vi "ADQUIRI_adq.vi"() -> ()   [LabVIEW 2019]
doc: "Programa que faz a leitura e a gravação em arquivo TXT de 13 canais provenientes da placa da National Instruments."
uses:
  <vilib>/DAQmx/read.llb/DAQmx Read (Analog 2D DBL NChan NSamp).vi
  <vilib>/Analysis/baseanly.llb/Mean (DBL).vi
  comunicacao.vi
  Aplicacao_atual_global_adq.vi
  <vilib>/DAQmx/configure/timing.llb/DAQmx Timing (Sample Clock).vi
  <vilib>/DAQmx/miscellaneous.llb/DAQmx Fill In Error Info.vi
  <vilib>/Utility/file.llb/Write Delimited Spreadsheet (DBL).vi
  <vilib>/Analysis/NI_AALBase.lvlib
  <vilib>/Utility/file.llb/Read Delimited Spreadsheet (string).vi
  <vilib>/Utility/file.llb/Write Delimited Spreadsheet (string).vi
panel:
  in  "JK(N. Arquivo)":string
  in  "JW(N. Arquivo)":string
  out "data path":path
  out "arrayPbar":dbl[](array[numeric])
  out "Pbarometro":dbl format="%#.2g"
  in  "JG(N. Arquivo)":string
  out "P1-P2 VERDE":bool
  out "comunica funcionando":bool
  in  "Calibração":bool
  in  "COMUNICA":bool
  out "DAQmx Task Name":refnum<k21>
  in  "Visualizar":bool
  out "led viewing":bool
  out "Configuração":string
  in  "Pontos No Gráfico":dbl(knob)=497.5700948522667 scale=0.0..3000.0
  in  "Frequência":dbl=3000.0
  out "Ok":bool
  out "OK2":bool
  out "Ok R":bool
  out "OK2 R":bool
  out "SKM-AI-KF-COR":dbl
  out "SKM-FI-WF":dbl format="%#.2g"
  out "SKM-FIC-KF-COR":dbl format="%#.2g"
  in  "SAIR":bool
  out "JG(m/s)":dbl
  in  "TempoAquisicao":dbl=60.0
  out "JW(m/s)":dbl format="%#.6g"
  out "JK(m/s)":dbl format="%#.6g"
  out "Timer":i32 caption="Elapsed Time (s)"
  in  "COMEÇAR":bool
  out "Quantidade de\narquivos adquiridos":i64
  out "LED adquiri":bool
  out "Aquisição Automática":bool
  out "Linha de Teste":bool
  in  "Tab Control":enum32{"Gráfico", "Matriz"}(tab)
  out "Aplicação":string
  in  "Help":bool
  out "Gráfico":dbl[][](graph)
  out "C1-M corrente":dbl format="%#_4g"
  out "C1-J corrente":dbl format="%#_4g"
  out "C2-M corrente":dbl format="%#_4g"
  out "C2-J corrente":dbl format="%#_4g"
  out "C3-M corrente":dbl format="%#_4g"
  out "C3-J corrente":dbl format="%#_4g"
  out "C4-M corrente":dbl format="%#_4g"
  out "C4-J corrente":dbl format="%#_4g"
  out "P1 corrente":dbl format="%#_4g"
  out "P2 corrente":dbl format="%#_4g"
  out "P3 corrente":dbl format="%#_4g"
  out "P4 corrente":dbl format="%#_4g"
  out "Pfundo corrente":dbl format="%#_4g"
  out "P4(kPa)":dbl format="%#.2g"
  out "P3(kPa)":dbl format="%#.2g"
  out "P2(kPa)":dbl format="%#.2g"
  out "P1(kPa)":dbl format="%#.2g"
  out "Pfundo(kPa)":dbl format="%#.2g"
  out "P4":dbl format="%#_2g"
  out "C4-J":dbl format="%#_2g"
  out "C4-M":dbl format="%#_2g"
  out "C3-J":dbl format="%#_2g"
  out "P3":dbl format="%#_2g"
  out "C3-M":dbl format="%#_2g"
  out "Pfundo":dbl format="%#_2g"
  out "C2-J":dbl format="%#_2g"
  out "P2":dbl format="%#_2g"
  out "C2-M":dbl format="%#_2g"
  out "P1":dbl format="%#_2g"
  out "C1-M":dbl format="%#_2g"
  out "C1-J":dbl format="%#_2g"
  out "Matriz":dbl[][](array[numeric])
  out "Finalizado":bool
  out "Aquisição":bool
  out "Visualização":bool
  out "Comunicação":bool
  in  "ValoresEnviados":T1
  out "SKS-NC-CV-006":bool
  in  "Valores":T2
  out "P1-P2 RED":bool
  out "P2-P3 RED":bool
  out "P3-P4 RED":bool
  out "P34/L [Pa/m]":dbl
  out "P23/L [Pa/m]":dbl
  out "P12/L [Pa/m]":dbl
  out "Valor Teórico[Pa/m]":dbl
  out "P3-P4 VERDE":bool
  out "P2-P3 VERDE":bool
  out "Valvulas":T3
  out "VALORES UDP":string[](array[string])
  out "reference out":refnum<vi>
  out "error out":errorcluster
  in  "SKM-AI-KF_CORIOLI [kg/m³]":dbl
  in  "SKM-FIC-KF_CORIOLI [kg/s]":dbl
  in  "SIW-CV-001":bool
  in  "SIK-CV-001":bool
  in  "Entrada - SKM-FI-WF [CLP]":dbl
  in  "Escala de Calibracao - SKM-FI-WF":cluster{"Escala Max":dbl, "Escala Min":dbl}
  # "<- Aquisição"
  # "[Hz]"
  # "Aquisição"
  # "[s]"
  # "m/s"
  # "m³/s"
  # "CHECK-UP"
  # "[s]"
  # "m/s"
  # "kg/s"
  # "P1, P3 & P4"
  # "kg/m³"
  # "P2"
  # "[mA]"
  # "[V]"
  # "[mA]"
  # "[V]"
  # "[mA]"
  # "[V]"
  # "[kPa]"
  # "[mA]"
  # "[V]"
  # "[mA]"
  # "[V]"
  # "[mA]"
  # "[V]"
  # "[kPa]"
  # "[mA]"
  # "[V]"
  # "[mA]"
  # "[V]"
  # "[mA]"
  # "[V]"
  # "[kPa]"
  # "[mA]"
  # "[V]"
  # "[mA]"
  # "[V]"
  # "[mA]"
  # "[V]"
  # "[kPa]"
  # "[mA]"
  # "[V]"
  # "[kPa]"
  # "MIN"
  # "MAX"
  # "P1"
  # "kPa"
  # "P2"
  # "kPa"
  # "P3"
  # "kPa"
  # "P4"
  # "kPa"
  # "Pfundo"
  # "kPa"
  # "Variáveis Selecionadas Para Aquisição"
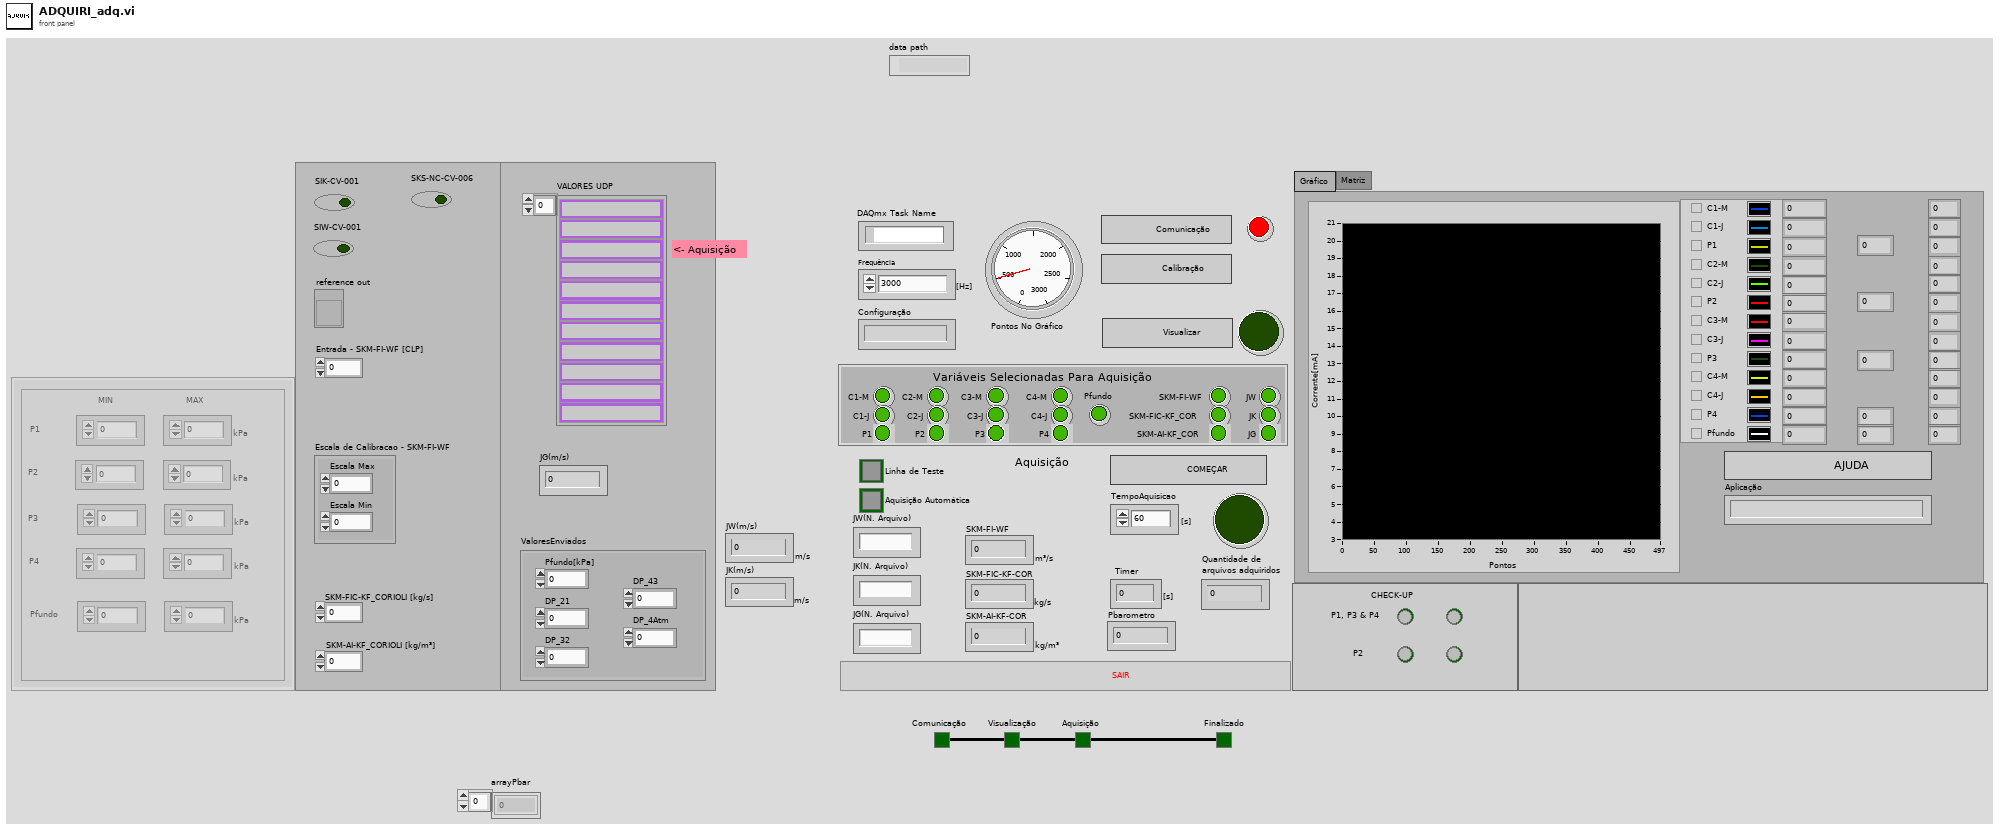
[diagram p1: front panel]
types:
  T1 = cluster{"Pfundo[kPa]":dbl, "DP_21":dbl, "DP_32":dbl, "DP_43":dbl, "DP_4Atm":dbl}
  T2 = cluster{"P1 MIN":i32, "P1 MAX":i32, "P2 MIN":i32, "P2 MAX":i32, "P3 MIN":i32, "P3 MAX":i32, "P4 MIN":i32, "P4 MAX":i32, "Pfu MIN":i32, "Pfu MAX":i32}
  T3 = cluster{"C1-M":bool, "C1-J":bool, "P1":bool, "C2-M":bool, "C2-J":bool, "P2":bool, "C3-M":bool, "C3-J":bool, "P3":bool, "C4-M":bool, "C4-J":bool, "P4":bool, "Pfundo":bool, "JW":bool, "JK":bool, "JG":bool, "SKM-FI-WF":bool, "SKM-FIC-KF_COR":bool, "SKM-AI-KF_COR":bool}
  T4 = enum8{"Enabled", "Disabled", "Disabled and Grayed Out"}
  T5 = enum32{"Invalid", "Standard", "Closed", "Hidden", "Minimized", "Maximized"}
  T6 = enum32{"Bad", "Idle", "Run top level", "Running"}
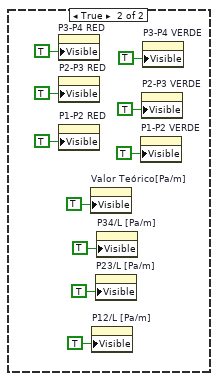
[diagram p3: hidden frame]
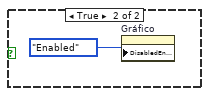
[diagram p5: hidden frame]
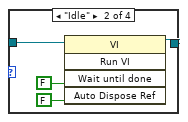
[diagram p6: hidden frame]
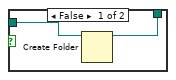
[diagram p9: hidden frame]
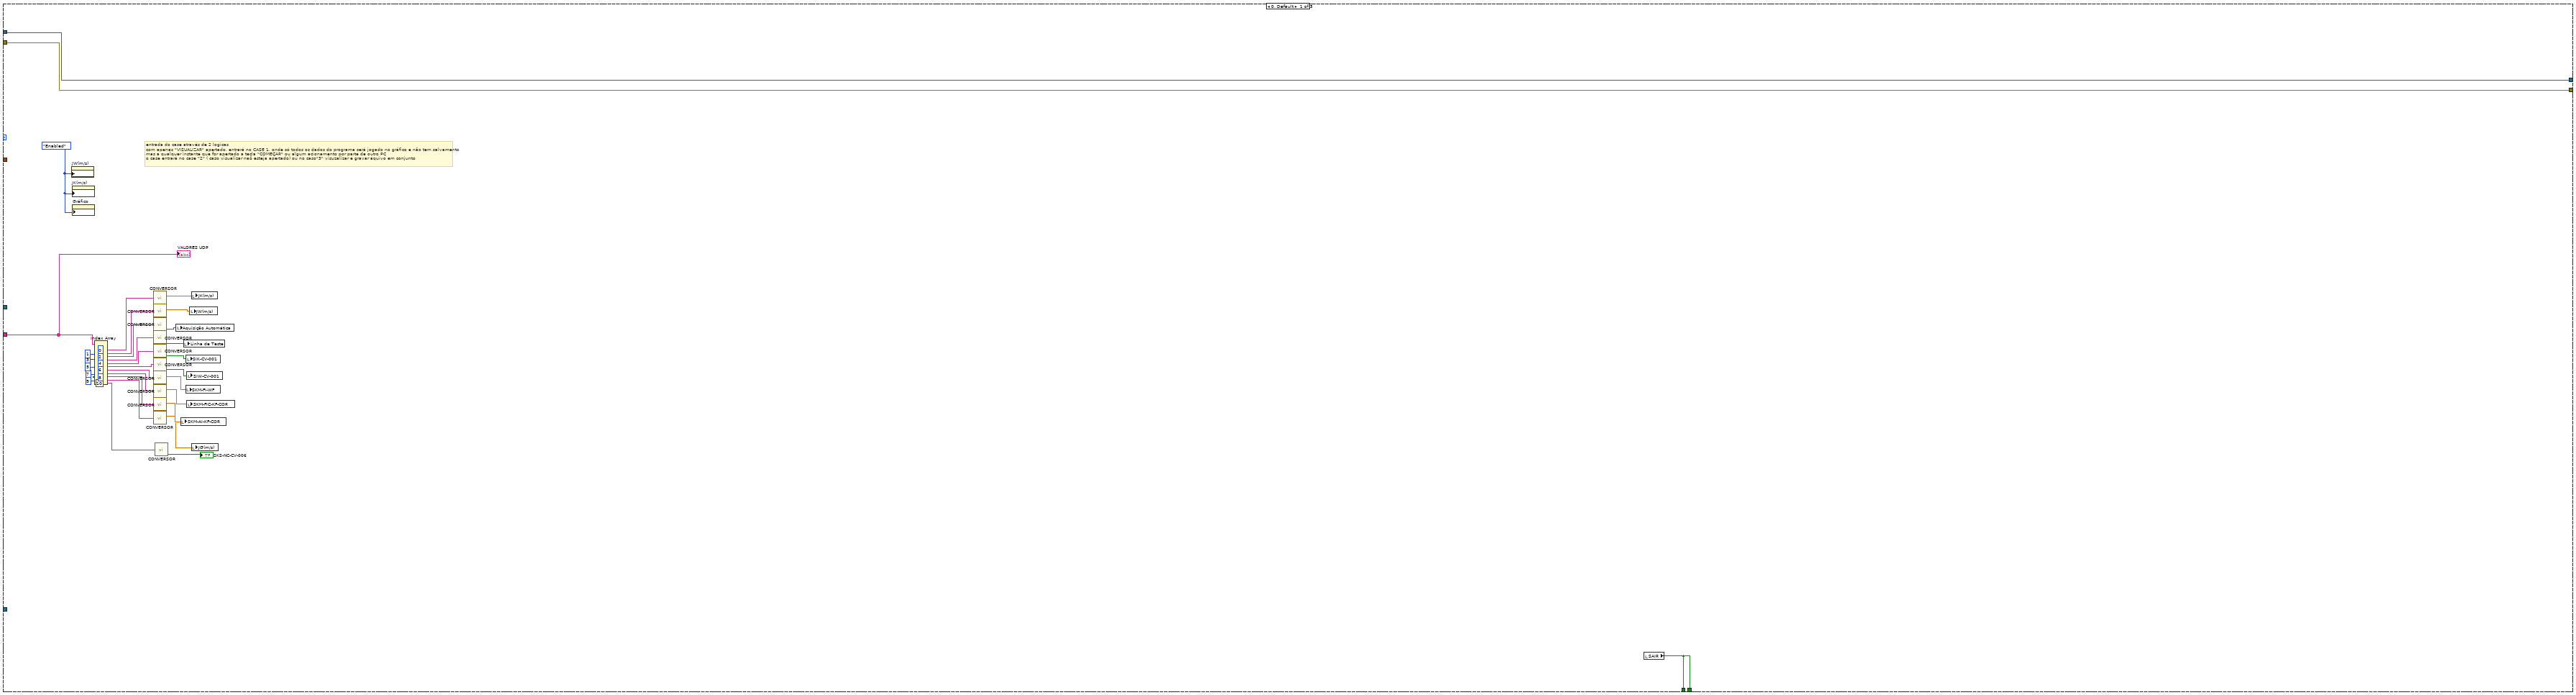
[diagram p10: hidden frame]
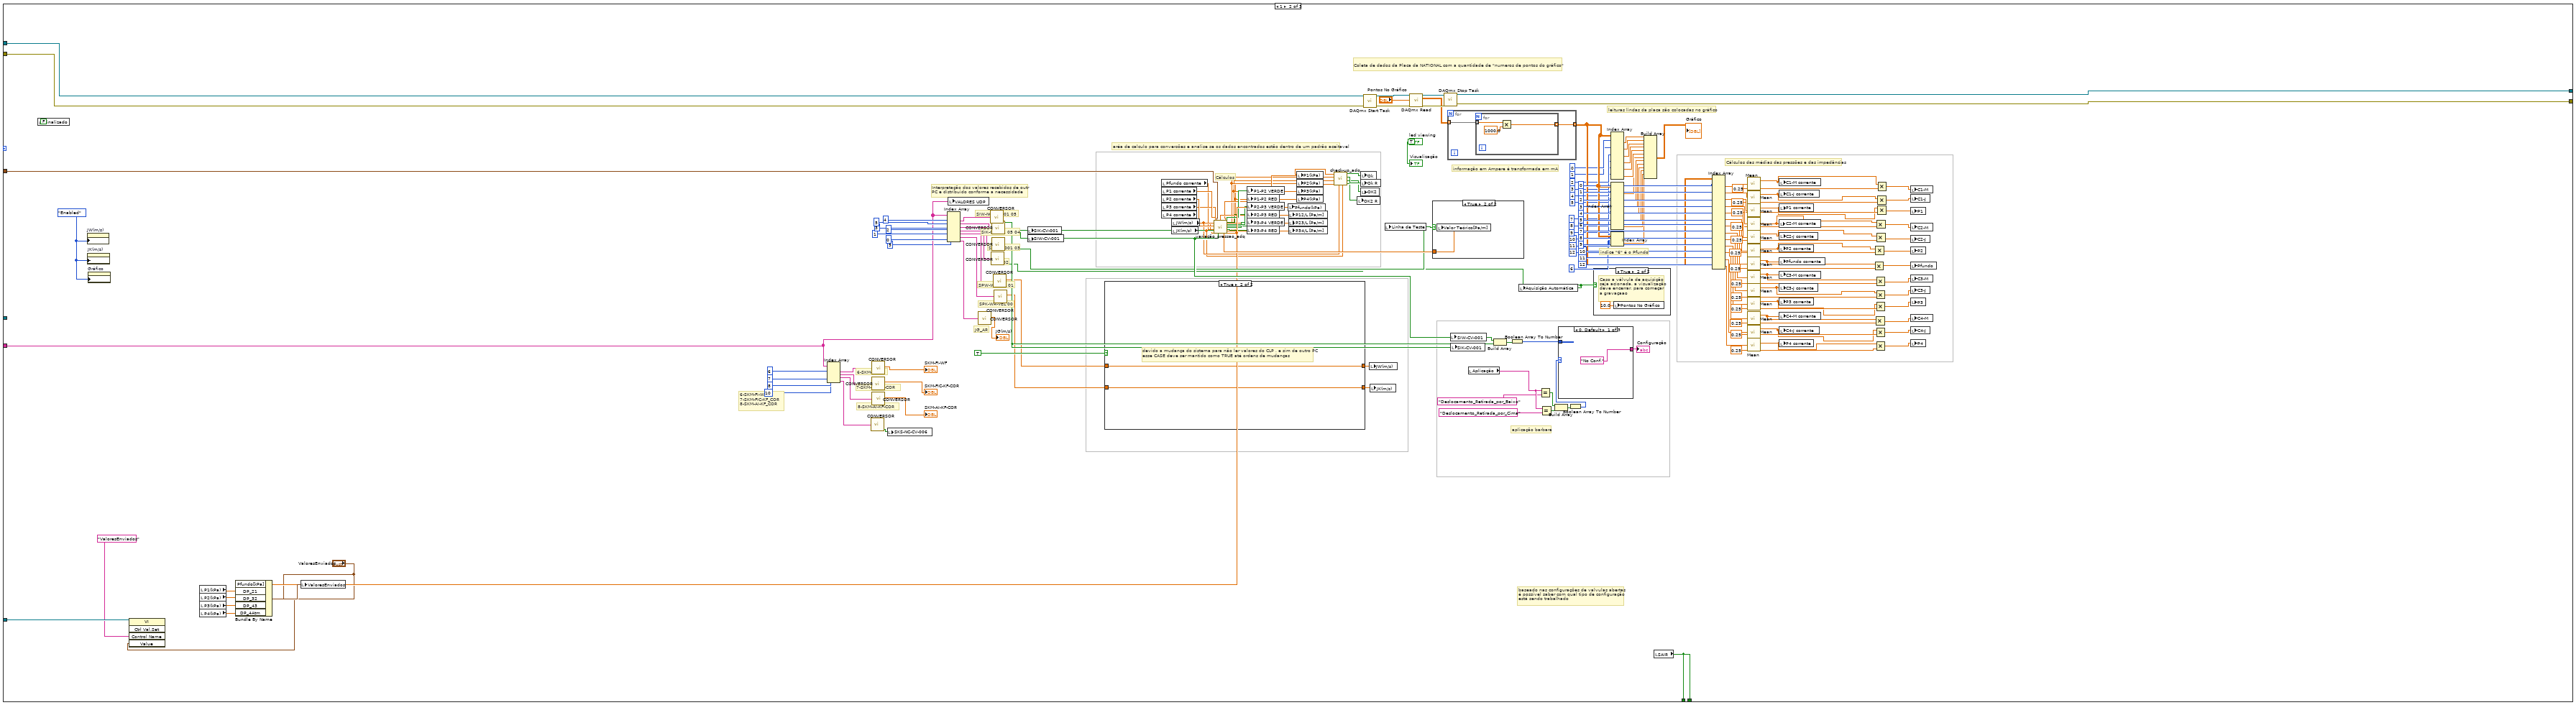
[diagram p11: hidden frame]
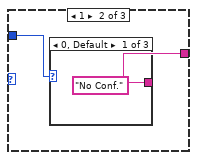
[diagram p12: hidden frame]
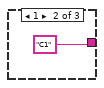
[diagram p13: hidden frame]
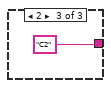
[diagram p14: hidden frame]
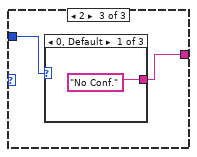
[diagram p15: hidden frame]
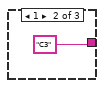
[diagram p16: hidden frame]
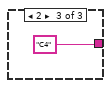
[diagram p17: hidden frame]
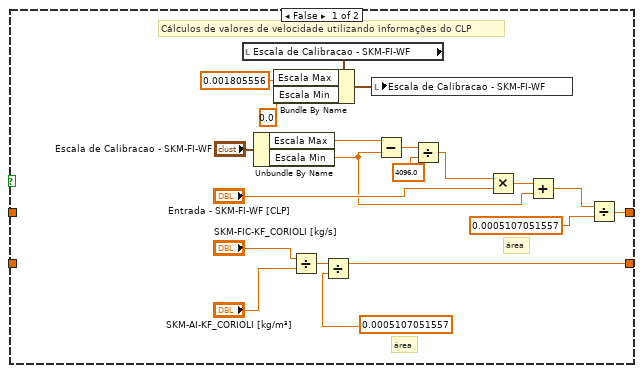
[diagram p18: hidden frame]
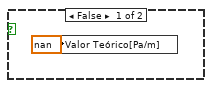
[diagram p20: hidden frame]
diagram:
  # "Abre a VI"
  n1 = property class="VI"("Front Panel.Open"=TRUE ("Front Panel Window:Open")) -> (error out=w1:errorcluster)  [unwired: 2 in, 1 out]
  n2 = flat-sequence {
    tunnel: [w5] -> w3
    tunnel: w1 -> [w4]
    tunnel: w3 -> [w730]
    frame #0 {
      n3 = while {
        shift-right: [w8] -> w5
        shift-left: w4 -> [w7]
        stop <- w6 stop-if-true
        # "Loop responsável\npor manter o \nadquiri rodando\n\nmesmo após uma \naquisição ou \nvisualização dos \ndados\no adquiri não irá\nfechar, e irá \naguardar um novo\ncomando"
        n4 = stacked-sequence {
          tunnel: [w29 _ _ _] -> w8
          tunnel: w7 -> [w29 _ _ _]
          tunnel: [_ _ _ w723] -> w6
          frame #0 {
            w20 = FALSE ("Visualisa")
            w9 = FALSE ("Visualisa")
            w33 = 0.0 ("element")
            # "aplicação barbara"
            # "Nessa parte do cógido, procuramos na aplicação atual, o seu diretório de armazenamento de dados, chamado\n\"DADOS\", cria-o se o mesmo n existir, caso exista, irá retornar a quantidade de arquivos ja adquiridos"
            # "Vi lê as configurações já definidas da aplicação atual e coloca na vairável\n\"VALVULAS\" para facilitar o manuzeio nesse programa"
            # "nessa parte do código , para o ADQUIRI teer acesso a algumas informações do CLP\no computador ADQUIRI evita de comunicar com o CLP para evitar erros futuros, então ele\npega as informações do computador SuperTorre, que é responsável por tratar esses dados\nnessa parte do código, procuramos o diretório UDP e colocamos para rodar o programa\n\"CLIENTE GERAL\" que será responsável por receber as informações do outro PC que contém\no programa\" SERVER GERAL\""
            # "Primeria parte da sequencia  do adquiri, inicia com todas as \nconfigurações e controle em seus estados default\nmatriz de armazenamento com até 17 posições para \narmazenamento de dados e transcrissão para o arquivo txt \nno final da sequencia\npontos no grafico com visualização de 3000 pontos por \nsegundo\ntempo de aquisição inicializado em 30 segundos, mas pode \nser alterado conforme a preferÊncia do usuário\nTimer inicia em 0, que será o tempo atual de aquisição\na configuração da aplicação inicia em default , pois ao longo \ndos acionamento do supervisório, irá saber de qual \nconfiguração se trata\ncontrole de pontos no gráfico encontra ativado\n\nem verde, temos todos os booleanos que necessitam ser\ninicializados em FALSE"
            # "Variáveis que precisam começar com valores iniciais"
            # "indicadores que precisam iniciar desligados"
            n5 = global read "Aplicacao_atual_global_adq.vi" "APLICACAO ATUAL"() -> (w10:string)
            "Aplicação" <- w10
            n6 = flat-sequence {
              frame #0 {
                n7 = global read "comunicacao.vi" "comunicacao"() -> (w55:bool)
                n8 = case shown="False" w55 {
                  frame False {
                    n9 = while {
                      stop <- w56 stop-if-true
                      n10 = One Button Dialog(message="LIGUE O SERVER E \nAPÓS ISSO,\n LIGAR COMUNICAÇÃO", button name ("OK")="OK") -> (true=w56:bool)
                    }
                  }
                  frame True {
                  }
                }
              }
              frame #1 {
                n11 = global read "comunicacao.vi" "comunicacao"() -> (w59:bool)
                n12 = case shown="False" w59 {
                  frame False {
                    n13 = while {
                      stop <- "COMUNICA" stop-if-true
                      n14 = property on="Gráfico" class="WFGraph (strict)"("DisabledEnum"=T4."Disabled and Grayed Out" ("Disabled")) -> ()  [unwired: 2 in, 2 out]
                    }
                  }
                  frame True {
                    n15 = property on="Gráfico" class="WFGraph (strict)"("DisabledEnum"=T4."Enabled" ("Disabled")) -> ()  [unwired: 2 in, 2 out]
                  }
                }
              }
              frame #2 {
                n16 = Current VI's Path() -> (path=w68:path)
                n17 = Strip Path(path=w68) -> (stripped path=w69:path)  [unwired: 1 out]
                n18 = Strip Path(path=w69) -> (stripped path=w70:path)  [unwired: 1 out]
                n19 = Build Path(base path=w70, name or relative path="UDP\\CLIENTE GERAL.vi") -> (appended path=w71:path)
                n20 = Open VI Reference(vi path=w71) -> (vi reference=w64:refnum<vi>)  [unwired: 5 in, 1 out]
                n21 = property class="VI"(reference=w64) -> (reference out=w65:refnum<vi>, "Exec.State"=w66:T6)  [unwired: 1 in, 1 out]
                n22 = case shown="\"Bad\", Default" w66 {
                  tunnel: w65 -> [w72 w74 w77 w78]
                  tunnel: [w72 w73 w77 w78] -> w63
                  frame "Bad", Default {
                  }
                  frame "Idle" {
                    n23 = invoke class="VI" method="Run VI"(reference=w74, "Wait until done"=FALSE ("Wait Until Done"), "Auto Dispose Ref"=FALSE ("Auto Dispose Reference")) -> (reference out=w73:refnum<vi>)  [unwired: 2 in, 4 out]
                  }
                  frame "Run top level" {
                  }
                  frame "Running" {
                  }
                }
                "reference out" <- w63
              }
            }
            n24 = Current VI's Path() -> (path=w28:path)
            n25 = Strip Path(path=w28) -> (stripped path=w27:path)  [unwired: 1 out]
            n26 = Equal?(x=w10, y="Deslocamento_Retirada_por_Baixo") -> (x = y?=w17:bool)
            n27 = Equal?(x=w10, y="Deslocamento_Retirada_por_Cima") -> (x = y?=w16:bool)
            n28 = Or(x=w17, y=w16) -> (x .or. y?=w15:bool)
            n29 = Build Path(base path=w27, name or relative path="PosProcessamento_UDP_NI\\data") -> (appended path=w23:path)
            n30 = property on="Pontos No Gráfico" class="Knob (strict)"("DisabledEnum"=T4."Enabled" ("Disabled")) -> ()  [unwired: 2 in, 2 out]
            n31 = property on="Calibração" class="Bool (strict)"("DisabledEnum"=T4."Enabled" ("Disabled")) -> ()  [unwired: 2 in, 2 out]
            n32 = Initialize Array(w33, w33, 16.0 ("element")) -> (→"Matriz":dbl[][])
            n33 = local write "Configuração"("No Conf." ("Configuration")) -> ()
            n34 = case shown="False" w15 {
              frame False {
                n35 = property on="P3-P4 RED" class="Bool (strict)"("Visible"=FALSE) -> ()  [unwired: 2 in, 2 out]
                n36 = property on="P2-P3 RED" class="Bool (strict)"("Visible"=FALSE) -> ()  [unwired: 2 in, 2 out]
                n37 = property on="P1-P2 RED" class="Bool (strict)"("Visible"=FALSE) -> ()  [unwired: 2 in, 2 out]
                n38 = property on="P1-P2 VERDE" class="Bool (strict)"("Visible"=FALSE) -> ()  [unwired: 2 in, 2 out]
                n39 = property on="P2-P3 VERDE" class="Bool (strict)"("Visible"=FALSE) -> ()  [unwired: 2 in, 2 out]
                n40 = property on="P3-P4 VERDE" class="Bool (strict)"("Visible"=FALSE) -> ()  [unwired: 2 in, 2 out]
                n41 = property on="P12/L [Pa/m]" class="DigNum (strict)"("Visible"=FALSE) -> ()  [unwired: 2 in, 2 out]
                n42 = property on="P23/L [Pa/m]" class="DigNum (strict)"("Visible"=FALSE) -> ()  [unwired: 2 in, 2 out]
                n43 = property on="P34/L [Pa/m]" class="DigNum (strict)"("Visible"=FALSE) -> ()  [unwired: 2 in, 2 out]
                n44 = property on="Valor Teórico[Pa/m]" class="DigNum (strict)"("Visible"=FALSE) -> ()  [unwired: 2 in, 2 out]
              }
              frame True {
                n45 = property on="P3-P4 RED" class="Bool (strict)"("Visible"=TRUE) -> ()  [unwired: 2 in, 2 out]
                n46 = property on="P2-P3 RED" class="Bool (strict)"("Visible"=TRUE) -> ()  [unwired: 2 in, 2 out]
                n47 = property on="P1-P2 RED" class="Bool (strict)"("Visible"=TRUE) -> ()  [unwired: 2 in, 2 out]
                n48 = property on="Valor Teórico[Pa/m]" class="DigNum (strict)"("Visible"=TRUE) -> ()  [unwired: 2 in, 2 out]
                n49 = property on="P12/L [Pa/m]" class="DigNum (strict)"("Visible"=TRUE) -> ()  [unwired: 2 in, 2 out]
                n50 = property on="P23/L [Pa/m]" class="DigNum (strict)"("Visible"=TRUE) -> ()  [unwired: 2 in, 2 out]
                n51 = property on="P34/L [Pa/m]" class="DigNum (strict)"("Visible"=TRUE) -> ()  [unwired: 2 in, 2 out]
                n52 = property on="P1-P2 VERDE" class="Bool (strict)"("Visible"=TRUE) -> ()  [unwired: 2 in, 2 out]
                n53 = property on="P2-P3 VERDE" class="Bool (strict)"("Visible"=TRUE) -> ()  [unwired: 2 in, 2 out]
                n54 = property on="P3-P4 VERDE" class="Bool (strict)"("Visible"=TRUE) -> ()  [unwired: 2 in, 2 out]
              }
            }
            n55 = local write "Timer"(0.0 ("Timer")) -> ()
            n56 = call <vilib>:"Check if File or Folder Exists.vi"("path"=w23) -> ("file or folder exists?"=w26:bool, "dup path"=w25:path)  [unwired: 8 in, 1 out]
            n57 = case shown="True" w26 {
              tunnel: w25 -> [w80 w81]
              tunnel: [w79 w81] -> w24
              frame False {
                n58 = Create Folder(path (use dialog)=w80) -> (created path=w79:path)  [unwired: 2 in, 2 out]
              }
              frame True {
              }
            }
            n59 = File/Directory Info(path=w24) -> (size=w13:i64)  [unwired: 1 in, 6 out]
            n60 = local write "Visualização"(w9) -> ()
            n61 = local write "led viewing"(w9) -> ()
            n62 = local write "LED adquiri"(w9) -> ()
            n63 = local write "Visualizar"(w9) -> ()
            n64 = local write "P1-P2 VERDE"(w9) -> ()
            n65 = local write "P1-P2 RED"(w9) -> ()
            n66 = local write "P2-P3 VERDE"(w9) -> ()
            n67 = local write "P2-P3 RED"(w9) -> ()
            n68 = local write "P3-P4 VERDE"(w9) -> ()
            n69 = local write "P3-P4 RED"(w9) -> ()
            n70 = local write "COMEÇAR"(w9) -> ()
            n71 = local write "Help"(w9) -> ()
            n72 = local write "SAIR"(w9) -> ()
            n73 = local write "Aquisição Automática"(w9) -> ()
            n74 = local write "comunica funcionando"(w9) -> ()
            n75 = local write "Comunicação"(w9) -> ()
            n76 = local write "Aquisição"(w9) -> ()
            n77 = Decrement(x=w13) -> (x-1=→"Quantidade de\narquivos adquiridos":i64)
            n78 = local write "Ok"(w20) -> ()
            n79 = local write "Ok R"(w20) -> ()
            n80 = local write "OK2"(w20) -> ()
            n81 = local write "OK2 R"(w20) -> ()
            n82 = call "leitura_configuracao_valvulas_adq.vi"() -> ("Valvulas"=→"Valvulas":T3)  [unwired: 6 in]
          }
          frame #1 {
            # "nessa etapa do programa, pegamos as referências dessas Vi\n\"LEITURA VALORES CLIENTE\" E \"CLIENTE GERAL\" que JÁ ESTÃO\nRODANDO EM OFF\ncom as refências em mãos, iremos jagá-las para dentro do loop"
            n83 = Current VI's Path() -> (path=w96:path)
            n84 = Current VI's Path() -> (path=w107:path)
            n85 = Strip Path(path=w107) -> (stripped path=w108:path)  [unwired: 1 out]
            n86 = Strip Path(path=w96) -> (stripped path=w90:path)  [unwired: 1 out]
            n87 = Strip Path(path=w108) -> (stripped path=w85:path)  [unwired: 1 out]
            n88 = Build Path(base path=w90, name or relative path="calibracao_adq.vi") -> (appended path=w94:path)
            n89 = Build Path(base path=w85, name or relative path="UDP\\ENVIA VALORES-CLIENTE.vi") -> (appended path=w84:path)
            n90 = Build Path(base path=w85, name or relative path="UDP\\LEITURA VALORES CLIENTE.vi") -> (appended path=w109:path)
            n91 = Build Path(base path=w85, name or relative path="UDP\\CLIENTE GERAL.vi") -> (appended path=w104:path)
            n92 = Open VI Reference(vi path=w84) -> (vi reference=w82:refnum<vi>)  [unwired: 5 in, 1 out]
            n93 = Open VI Reference(vi path=w94, error in (no error)=errorcluster {"status"=FALSE, "code"=0, "source"=""}) -> (vi reference=w93:refnum<vi>, error out=w92:errorcluster)  [unwired: 4 in]
            n94 = Open VI Reference(vi path=w109) -> (vi reference=w105:refnum<vi>)  [unwired: 5 in, 1 out]
            n95 = Open VI Reference(vi path=w104) -> (vi reference=w102:refnum<vi>)  [unwired: 5 in, 1 out]
            n96 = invoke class="VI" method="Run VI"(reference=w93, error in=w92, "Wait until done"=FALSE ("Wait Until Done"), "Auto Dispose Ref"=TRUE ("Auto Dispose Reference")) -> (reference out=w98:refnum<vi>, error out=w97:errorcluster)  [unwired: 1 in, 3 out]
            n97 = invoke class="VI" method="Ctrl Val.Get"(reference=w98, error in=w97, "Control Name"="Valores") -> (reference out=w88:refnum<vi>, error out=w87:errorcluster, "Get Control Value Variant"=w86:variant)  [unwired: 1 in, 1 out]
            n98 = while {
              tunnel: w105 -> [w123]
              tunnel: w102 -> [w146]
              shift-right: [w136] -> w89
              shift-left: w88 -> [w132]
              shift-right: [w135] -> _
              shift-left: w87 -> [w133]
              shift-right: [w131] -> _
              shift-left: w86 -> [w134]
              tunnel: w82 -> [w124]
              stop <- w158 stop-if-true
              w121 = refnum<k21> "ADQUIRE" ("DAQmx Task Name")
              w120 = 10123 items=["Finite Samples"=10178, "Continuous Samples"=10123, "Hardware Timed Single Point"=12522] ("sample mode")
              w111 = FALSE ("visu led")
              # "11"
              # "Parte de comunicação com a placa da NATIONAL\nINSTRUMENTS\nno módulo de comunicação chamado DAQmx\nselecionamos o tipo \"continuous SAMPLES\" para a\ncoleta de amostras contínuas\ntambém entramos com o nome de TASK chamado\nADQUIRE, que já contém informações de leitura \njá pré programadas\nFrequência padrão de 3000Hz"
              # "10"
              # "9"
              # "8"
              # "7"
              # "6"
              # "5"
              # "4"
              # "3"
              # "2"
              # "1"
              # "0"
              # "acionamento automático recebido de outro\nPC"
              # "Default dos botões"
              # "Caso as configurações não desejam\nincluir alguma velocidade na aquisição\na mesma será desabilitada"
              # "Coleta os valores das variáveis enviadas abaixo\nos valores são devolvidos na mesma ordem"
              # "Envia para o programa de comunicação com o outro computador\numa lista de nomes de variáveis que o ADQUIRE nessecita \nos nomes precisam ser enviados em array de STRING para o funcionamento\ndo programa de comunicação."
              # "ADQ 02"
              n99 = local read "Valvulas"() -> (w150:T3)
              n100 = local write "Ok R"(w111) -> ()
              n101 = local write "Visualização"(w111) -> ()
              n102 = local write "led viewing"(w111) -> ()
              n103 = local write "OK2"(w111) -> ()
              n104 = local write "OK2 R"(w111) -> ()
              n105 = local write "Ok"(w111) -> ()
              n106 = case shown="True" "Help" {
                frame False {
                  # "Botão Help destinado a abrir documentos e pesquisas relacionadas\nele também abre uma janela explicando sucintamente o objetivo do \nprograma ADQUIRE"
                }
                frame True {
                  n107 = stacked-sequence {
                    frame #0 {
                      n108 = Current VI's Path() -> (path=w678:path)
                      n109 = Current VI's Path() -> (path=w672:path)
                      n110 = Strip Path(path=w678) -> (stripped path=w677:path)  [unwired: 1 out]
                      n111 = Strip Path(path=w672) -> (stripped path=w671:path)  [unwired: 1 out]
                      n112 = Build Path(base path=w677, name or relative path="Help_difinicao_adq.vi") -> (appended path=w675:path)
                      n113 = Build Path(base path=w671, name or relative path="help_pdfs_adq.vi") -> (appended path=w669:path)
                      n114 = Open VI Reference(vi path=w675) -> (vi reference=w682:refnum<vi>, error out=w681:errorcluster)  [unwired: 5 in]
                      n115 = Open VI Reference(vi path=w669) -> (vi reference=w680:refnum<vi>, error out=w679:errorcluster)  [unwired: 5 in]
                      n116 = invoke class="VI" method="Run VI"(reference=w682, error in=w681, "Wait until done"=FALSE ("Wait Until Done"), "Auto Dispose Ref"=FALSE ("Auto Dispose Reference")) -> ()  [unwired: 1 in, 5 out]
                      n117 = invoke class="VI" method="Run VI"(reference=w680, error in=w679, "Wait until done"=FALSE ("Wait Until Done"), "Auto Dispose Ref"=FALSE ("Auto Dispose Reference")) -> ()  [unwired: 1 in, 5 out]
                    }
                    frame #1 {
                      n118 = local write "Help"(FALSE ("Help")) -> ()
                    }
                  }
                }
              }
              n119 = Unbundle By Name(w150) -> ("JW"=w151:bool, "JK"=w152:bool, "JG"=w153:bool)
              n120 = case shown="True" w151 {
                frame False {
                  n121 = property on="JW(m/s)" class="DigNum (strict)"("DisabledEnum"=T4."Disabled and Grayed Out" ("Disabled")) -> ()  [unwired: 2 in, 2 out]
                }
                frame True {
                  n122 = property on="JW(m/s)" class="DigNum (strict)"("DisabledEnum"=T4."Enabled" ("Disabled")) -> ()  [unwired: 2 in, 2 out]
                }
              }
              n123 = case shown="True" w152 {
                frame False {
                  n124 = property on="JK(m/s)" class="DigNum (strict)"("DisabledEnum"=T4."Disabled and Grayed Out" ("Disabled")) -> ()  [unwired: 2 in, 2 out]
                }
                frame True {
                  n125 = property on="JK(m/s)" class="DigNum (strict)"("DisabledEnum"=T4."Enabled" ("Disabled")) -> ()  [unwired: 2 in, 2 out]
                }
              }
              n126 = case shown="True" w153 {
                frame False {
                  n127 = property on="JG(m/s)" class="DigNum (strict)"("DisabledEnum"=T4."Disabled and Grayed Out" ("Disabled")) -> ()  [unwired: 2 in, 2 out]
                }
                frame True {
                  n128 = property on="JG(m/s)" class="DigNum (strict)"("DisabledEnum"=T4."Enabled" ("Disabled")) -> ()  [unwired: 2 in, 2 out]
                }
              }
              n129 = case shown="False" "Calibração" {
                tunnel: [w642 w650] -> w136
                tunnel: [w643 w649] -> w135
                tunnel: [w644 w648] -> w131
                tunnel: w132 -> [w641 w647]
                tunnel: w133 -> [w640 w646]
                tunnel: w134 -> [_ _]
                frame False {
                  n130 = invoke class="VI" method="Ctrl Val.Get"(reference=w641, error in=w640, "Control Name"="Valores") -> (reference out=w642:refnum<vi>, error out=w643:errorcluster, "Get Control Value Variant"=w644:variant)  [unwired: 1 in, 1 out]
                }
                frame True {
                  n131 = stacked-sequence {
                    tunnel: [w655 _] -> w650
                    tunnel: [w654 _] -> w649
                    tunnel: [w653 _] -> w648
                    tunnel: w647 -> [w652 _]
                    tunnel: w646 -> [w651 _]
                    frame #0 {
                      n132 = invoke class="VI" method="FP.Open"(reference=w652, error in=w651, "State"=T5."Standard") -> (reference out=w657:refnum<vi>, error out=w656:errorcluster)  [unwired: 2 in, 3 out]
                      n133 = invoke class="VI" method="Ctrl Val.Get"(reference=w657, error in=w656, "Control Name"="Valores") -> (reference out=w655:refnum<vi>, error out=w654:errorcluster, "Get Control Value Variant"=w653:variant)  [unwired: 1 in, 1 out]
                    }
                    frame #1 {
                      n134 = local write "Calibração"(FALSE ("Calibração")) -> ()
                    }
                  }
                }
              }
              n135 = invoke class="VI" method="Ctrl Val.Get"(reference=w123, "Control Name"="VALORES") -> ("Get Control Value Variant"=w149:variant)  [unwired: 2 in, 3 out]
              n136 = property on="Gráfico" class="WFGraph (strict)"("DisabledEnum"=T4."Enabled" ("Disabled")) -> ()  [unwired: 2 in, 2 out]
              n137 = Variant To Data(type=string[] [] ("Array"), Variant=w149) -> (data=w128:string[])  [unwired: 1 in, 1 out]
              n138 = To Variant(anything=string[] ["JK", "JW", "ADQ", "SIT-NC-CV-001", "SIK-NC-CV-001", "SIW-NC-CV-001", "SKM-FI-WF", "SKM-FIC-KF_COR", "SKM-AI-KF_COR", "JG", "SKS-NC-CV-006", "SKM-PI-BAR"] ("NOMES")) -> (Variant=w141:variant)
              n139 = invoke class="VI" method="Ctrl Val.Set"(reference=w146, "Control Name"="NOMES", "Value"=w141) -> ()  [unwired: 2 in, 5 out]
              n140 = Index Array(array=w128, index=2) -> (element=w144:string)
              n141 = call "CONVERSOR.vi"("String"=w144) -> ("boolean"=w143:bool)  [unwired: 6 in, 3 out]
              "Aquisição Automática" <- w143
              n142 = Not Equal?(x=w128, y="") -> (x != y?=w127:bool[])
              n143 = Get Variant Attribute(Variant=w131, name="Valores") -> ()  [unwired: 2 in, 4 out]
              n144 = Variant To Data(type="Valores", Variant=w131) -> (data=w129:T2)  [unwired: 1 in, 1 out]
              n145 = Index Array(array=w127, index=0) -> (element=→"comunica funcionando" →"Comunicação":bool)
              n146 = local write "Valores"(w129) -> ()
              n147 = Or(x="COMEÇAR", y=w143) -> (x .or. y?=w155:bool)
              n148 = Build Array("Visualizar", w155) -> (w160:bool[])
              n149 = Boolean Array To Number(Boolean array=w160) -> (number=w159:u32)
              n150 = call-poly <vilib>:"DAQmx Timing.vi"("task/channels in"=w121, "sample mode"=w120, "rate"="Frequência", "source"=tag "OnboardClock") -> ("task out"=w118:refnum<k21>, "error out"=w117:errorcluster)  [unwired: 10 in]
              n151 = case shown="2, 3" w159 {
                tunnel: [w162 w229 w438] -> w157
                tunnel: [w162 w229 w437] -> w156
                tunnel: w128 -> [w196 w302 w436]
                tunnel: w118 -> [w198 w292 _]
                tunnel: w117 -> [w197 w291 _]
                tunnel: [w198 w290 w432] -> w115
                tunnel: [w197 w289 w433] -> w114
                tunnel: w129 -> [_ w246 w435]
                tunnel: w124 -> [_ w233 w434]
                tunnel: w123 -> [_ _ w431]
                frame 0, Default {
                  w161 = T4."Enabled" ("Disabled")
                  # "entrada do case através de 2 logicas\ncom apenas \"VISUALIZAR\" apertado, entrará no CASE 1, onde só todos os dados do programa será jogado no gráfico e não tem salvamento\nmas a qualquer instante que for apertado a tecla \"COMEÇAR\" ou algum acionamento por parte de outro PC\no case entrará no case \"2\" ( caso visualizar naõ esteja apertado) ou no caso\"3\" visuzalizar e gravar aquivo em conjunto"
                  n152 = property on="JW(m/s)" class="DigNum (strict)"("DisabledEnum"=w161) -> ()  [unwired: 2 in, 2 out]
                  n153 = property on="JK(m/s)" class="DigNum (strict)"("DisabledEnum"=w161) -> ()  [unwired: 2 in, 2 out]
                  n154 = property on="Gráfico" class="WFGraph (strict)"("DisabledEnum"=w161) -> ()  [unwired: 2 in, 2 out]
                  n155 = Index Array(array=w196, index #1=0 ("index"), index #2=1 ("index"), index #3=2 ("index"), index #4=3 ("index"), index #5=4 ("index"), index #6=5 ("index"), index #7=6 ("index"), index #8=7 ("index"), index #9=8 ("index"), index #10=9 ("index"), index #11=10 ("index")) -> (element #1=w185:string, element #2=w184:string, element #3=w183:string, element #4=w182:string, element #5=w181:string, element #6=w180:string, element #7=w179:string, element #8=w178:string, element #9=w177:string, element #10=w176:string, element #11=w165:string)
                  n156 = call "CONVERSOR.vi"("String"=w185) -> ("float"=w175:dbl)  [unwired: 6 in, 3 out]
                  n157 = call "CONVERSOR.vi"("String"=w184) -> ("float"=w174:dbl)  [unwired: 6 in, 3 out]
                  n158 = call "CONVERSOR.vi"("String"=w183) -> ("boolean"=w173:bool)  [unwired: 6 in, 3 out]
                  n159 = call "CONVERSOR.vi"("String"=w182) -> ("boolean"=w172:bool)  [unwired: 6 in, 3 out]
                  n160 = call "CONVERSOR.vi"("String"=w181) -> ("boolean"=w171:bool)  [unwired: 6 in, 3 out]
                  n161 = call "CONVERSOR.vi"("String"=w180) -> ("boolean"=w170:bool)  [unwired: 6 in, 3 out]
                  n162 = call "CONVERSOR.vi"("String"=w179) -> ("float"=w169:dbl)  [unwired: 6 in, 3 out]
                  n163 = call "CONVERSOR.vi"("String"=w178) -> ("float"=w168:dbl)  [unwired: 6 in, 3 out]
                  n164 = call "CONVERSOR.vi"("String"=w177) -> ("float"=w167:dbl)  [unwired: 6 in, 3 out]
                  n165 = call "CONVERSOR.vi"("String"=w176) -> ("float"=w166:dbl)  [unwired: 6 in, 3 out]
                  n166 = call "CONVERSOR.vi"("String"=w165) -> ("boolean"=→"SKS-NC-CV-006":bool)  [unwired: 6 in, 3 out]
                  n167 = local write "Aquisição Automática"(w173) -> ()
                  n168 = local write "SKM-AI-KF-COR"(w167) -> ()
                  n169 = local write "Linha de Teste"(w172) -> ()
                  n170 = local write "SKM-FI-WF"(w169) -> ()
                  n171 = local write "SIK-CV-001"(w171) -> ()
                  n172 = local write "SIW-CV-001"(w170) -> ()
                  n173 = local write "SKM-FIC-KF-COR"(w168) -> ()
                  n174 = local write "JW(m/s)"(w174) -> ()
                  n175 = local write "JK(m/s)"(w175) -> ()
                  n176 = local write "JG(m/s)"(w166) -> ()
                  n177 = local read "SAIR"() -> (w162:bool)
                  "VALORES UDP" <- w196
                }
                frame 1 {
                  w228 = T4."Enabled" ("Disabled")
                  w231 = TRUE ("visu led")
                  # "Cálculos"
                  # "aplicação barbara"
                  # "JG_AR"
                  # "6-SKM-FI-WF"
                  # "7-SKM-FIC-KF-COR"
                  # "8-SKM-AI-KF-COR"
                  # "6-SKM-FI-WF\n7-SKM-FIC-KF_COR\n8-SKM-AI-KF_COR"
                  # "indice \"6\" é o Pfundo"
                  # "leituras lindas da placa são colocadas no gráfico"
                  # "baseado nas configurações de valvulas abertas\né possível saber com qual tipo de configuração \nestá sendo trabalhado"
                  # "aréa de calculo para conversões e analise se os dados encontrados estão dentro de um padrão aceitavel"
                  # "Interpretação dos valores recebidos de outr\nPC e distribuido conforme a necessidade"
                  # "informação em Ampere é transformada em mA"
                  # "Coleta de dados da Placa da NATIONAL com a quantidade de \"numeros de pontos do gráfico\""
                  # "ADQ 02"
                  # "SIW-NC-CV-001 05"
                  # "SIK-CV-001 05 04"
                  # "SIT-CV-001 03"
                  # "SPW-WR-VEL 01"
                  # "SPK-WR-VEL 00"
                  # "Cálculos das médias das pressões e das impedâncias"
                  n178 = local write "Finalizado"(FALSE ("Finalizado")) -> ()
                  n179 = property on="JW(m/s)" class="DigNum (strict)"("DisabledEnum"=w228) -> ()  [unwired: 2 in, 2 out]
                  n180 = property on="JK(m/s)" class="DigNum (strict)"("DisabledEnum"=w228) -> ()  [unwired: 2 in, 2 out]
                  n181 = property on="Gráfico" class="WFGraph (strict)"("DisabledEnum"=w228) -> ()  [unwired: 2 in, 2 out]
                  n182 = invoke class="VI" method="Ctrl Val.Set"(reference=w233, "Control Name"="ValoresEnviados", "Value"="ValoresEnviados") -> ()  [unwired: 2 in, 5 out]
                  n183 = local read "P1(kPa)"() -> (w202:dbl)
                  n184 = local read "P2(kPa)"() -> (w201:dbl)
                  n185 = local read "P3(kPa)"() -> (w200:dbl)
                  n186 = local read "P4(kPa)"() -> (w199:dbl)
                  n187 = Index Array(array=w302, index #1=6 ("index"), index #2=7 ("index"), index #3=8 ("index"), index #4=10 ("index")) -> (element #1=w298:string, element #2=w297:string, element #3=w296:string, element #4=w244:string)
                  n188 = call "CONVERSOR.vi"("String"=w244) -> ("boolean"=w243:bool)  [unwired: 6 in, 3 out]
                  n189 = call "CONVERSOR.vi"("String"=w297) -> ("float"=→"SKM-FIC-KF-COR":dbl)  [unwired: 6 in, 3 out]
                  n190 = call "CONVERSOR.vi"("String"=w298) -> ("float"=→"SKM-FI-WF":dbl)  [unwired: 6 in, 3 out]
                  n191 = call "CONVERSOR.vi"("String"=w296) -> ("float"=→"SKM-AI-KF-COR":dbl)  [unwired: 6 in, 3 out]
                  n192 = local write "SKS-NC-CV-006"(w243) -> ()
                  n193 = Index Array(array=w302, index #1=4 ("index"), index #2=5 ("index"), index #3=3 ("index"), index #4=2 ("index"), index #5=1 ("index"), index #6=0 ("index"), index #7=9 ("index")) -> (element #1=w319:string, element #2=w318:string, element #3=w315:string, element #4=w311:string, element #5=w307:string, element #6=w304:string, element #7=w287:string)
                  n194 = local write "VALORES UDP"(w302) -> ()
                  n195 = call "CONVERSOR.vi"("String"=w287) -> ("float"=→"JG(m/s)":dbl)  [unwired: 6 in, 3 out]
                  n196 = call "CONVERSOR.vi"("String"=w319) -> ("boolean"=w313:bool)  [unwired: 6 in, 3 out]
                  n197 = call "CONVERSOR.vi"("String"=w311) -> ("boolean"=w310:bool)  [unwired: 6 in, 3 out]
                  n198 = call "CONVERSOR.vi"("String"=w318) -> ("boolean"=w317:bool)  [unwired: 6 in, 3 out]
                  n199 = call "CONVERSOR.vi"("String"=w315) -> ("boolean"=w314:bool)  [unwired: 6 in, 3 out]
                  n200 = call "CONVERSOR.vi"("String"=w307) -> ("float"=w306:dbl)  [unwired: 6 in, 3 out]
                  n201 = call "CONVERSOR.vi"("String"=w304) -> ("float"=w303:dbl)  [unwired: 6 in, 3 out]
                  n202 = local write "SIK-CV-001"(w313) -> ()
                  n203 = local write "SIW-CV-001"(w317) -> ()
                  n204 = case shown="True" TRUE {
                    tunnel: [w400 w419] -> w376
                    tunnel: [w399 w420] -> w375
                    tunnel: w306 -> [_ w420]
                    tunnel: w303 -> [_ w419]
                    frame False {
                      # "Cálculos de valores de velocidade utilizando informações do CLP"
                      # "área"
                      # "área"
                      n205 = local read "Escala de Calibracao - SKM-FI-WF"() -> (w406:cluster{"Escala Max":dbl, "Escala Min":dbl})
                      n206 = Unbundle By Name("Escala de Calibracao - SKM-FI-WF") -> ("Escala Max"=w409:dbl, "Escala Min"=w408:dbl)
                      n207 = Bundle By Name(cluster=w406, "Escala Max"=0.001805556, "Escala Min"=0.0 ("Escala Max")) -> (w407:cluster{"Escala Max":dbl, "Escala Min":dbl})
                      n208 = Divide(x="SKM-FIC-KF_CORIOLI [kg/s]", y="SKM-AI-KF_CORIOLI [kg/m³]") -> (x/y=w418:dbl)
                      n209 = Divide(x=w418, y=0.0005107051557) -> (x/y=w400:dbl)
                      n210 = local write "Escala de Calibracao - SKM-FI-WF"(w407) -> ()
                      n211 = Subtract(x=w409, y=w408) -> (x-y=w410:dbl)
                      n212 = Divide(x=w410, y=4096.0) -> (x/y=w411:dbl)
                      n213 = Multiply(x=w411, y="Entrada - SKM-FI-WF [CLP]") -> (x*y=w412:dbl)
                      n214 = Add(x=w412, y=w408) -> (x+y=w415:dbl)
                      n215 = Divide(x=w415, y=0.0005107051557) -> (x/y=w399:dbl)
                    }
                    frame True {
                      # "devido a mudança do sistema para não ler valores do CLP , e sim de outro PC\nesse CASE deve ser mantido como TRUE até ordens de mudanças"
                    }
                  }
                  n216 = local read "Pfundo corrente"() -> (w214:dbl)
                  n217 = local read "P1 corrente"() -> (w227:dbl)
                  n218 = local read "P2 corrente"() -> (w226:dbl)
                  n219 = local read "P3 corrente"() -> (w225:dbl)
                  n220 = local read "P4 corrente"() -> (w218:dbl)
                  n221 = local read "JW(m/s)"() -> (w205:dbl)
                  n222 = local read "JK(m/s)"() -> (w204:dbl)
                  n223 = call "variação_pressao_adq.vi"("P1(mA)"=w227, "P2(mA)"=w226, "P3(mA)"=w225, "P4(mA)"=w218, "PFUNDO(mA)"=w214, "JW(m/s)"=w205, "JK(m/s)"=w204, "Valores"=w246, "SIK-CV-001"=w313, "SIW-CV-001"=w317) -> ("P12/L12"=w219:dbl, "P34/L34"=w221:dbl, "P23/L23"=w220:dbl, "P2(kPa)"=w208:dbl, "VALOR TEORICO"=w380:dbl, "P3(kPa)"=w207:dbl, "P1(kPa)"=w209:dbl, "P4(kPa)"=w206:dbl, "P1-P2G"=w224:bool, "P2-P3R"=w215:bool, "P2-P3G"=w223:bool, "P1-P2R"=w217:bool, "P3-P4G"=w222:bool, "P3-P4R"=w216:bool, "PFUNDO(kPa)"=w234:dbl)  [unwired: 3 in]
                  n224 = Bundle By Name(cluster="ValoresEnviados", "Pfundo[kPa]"=w234, "DP_21"=w202, "DP_32"=w201, "DP_43"=w200, "DP_4Atm"=w199) -> (w235:T1)
                  n225 = local write "ValoresEnviados"(w235) -> ()
                  n226 = local write "P1-P2 VERDE"(w224) -> ()
                  n227 = local write "P1-P2 RED"(w217) -> ()
                  n228 = local write "P2-P3 VERDE"(w223) -> ()
                  n229 = local write "P2-P3 RED"(w215) -> ()
                  n230 = local write "P3-P4 VERDE"(w222) -> ()
                  n231 = local write "P3-P4 RED"(w216) -> ()
                  n232 = local write "Pfundo(kPa)"(w234) -> ()
                  n233 = local write "P12/L [Pa/m]"(w219) -> ()
                  n234 = local write "P23/L [Pa/m]"(w220) -> ()
                  n235 = local write "P34/L [Pa/m]"(w221) -> ()
                  n236 = local write "P1(kPa)"(w209) -> ()
                  n237 = local write "P2(kPa)"(w208) -> ()
                  n238 = local write "P3(kPa)"(w207) -> ()
                  n239 = local write "P4(kPa)"(w206) -> ()
                  n240 = call "check-up_adq.vi"("JK(m/s)"=w204, "JW(m/s)"=w205, "P4(kPa)"=w206, "P3(kPa)"=w207, "P2(kPa)"=w208, "P1(kPa)"=w209) -> ("OK 2 R"=w210:bool, "OK 2 G"=w211:bool, "OK RED"=w212:bool, "OK G"=w213:bool)  [unwired: 2 in]
                  n241 = local write "OK2 R"(w210) -> ()
                  n242 = local write "Ok"(w213) -> ()
                  n243 = local write "Ok R"(w212) -> ()
                  n244 = local write "OK2"(w211) -> ()
                  n245 = call <vilib>:"DAQmx Start Task.vi"("task/channels in"=w292, "error in"=w291) -> ("task out"=w387:refnum<k21>, "error out"=w386:errorcluster)  [unwired: 12 in]
                  n246 = local write "JW(m/s)"(w375) -> ()
                  n247 = local write "JK(m/s)"(w376) -> ()
                  n248 = local write "Linha de Teste"(w314) -> ()
                  n249 = call-poly <vilib>:"DAQmx Read.vi"("task/channels in"=w387, "number of samples per channel"="Pontos No Gráfico", "error in"=w386) -> ("task out"=w385:refnum<k21>, "data"=w383:dbl[][], "error out"=w384:errorcluster)  [unwired: 10 in]
                  n250 = case shown="True" w314 {
                    tunnel: w380 -> [_ w423]
                    frame False {
                      n251 = local write "Valor Teórico[Pa/m]"(nan) -> ()
                    }
                    frame True {
                      n252 = local write "Valor Teórico[Pa/m]"(w423) -> ()
                    }
                  }
                  n253 = call <vilib>:"DAQmx Stop Task.vi"("task/channels in"=w385, "error in"=w384) -> ("task out"=w290:refnum<k21>, "error out"=w289:errorcluster)  [unwired: 12 in]
                  n254 = for {
                    tunnel: w383 -> [w424] mode=indexing
                    tunnel: [w425] -> w349 mode=indexing
                    n255 = for {
                      tunnel: w424 -> [w428] mode=indexing
                      tunnel: [w426] -> w425 mode=indexing
                      n256 = Multiply(x=w428, y=1000.0) -> (x*y=w426:dbl)
                    }
                  }
                  n257 = local write "SIW-CV-001"(w317) -> ()
                  n258 = local write "SIK-CV-001"(w313) -> ()
                  n259 = local read "Aplicação"() -> (w242:string)
                  n260 = Build Array(w317, w313) -> (w377:bool[])
                  n261 = Boolean Array To Number(Boolean array=w377) -> (number=w379:u32)
                  n262 = local write "Aquisição Automática"(w310) -> ()
                  n263 = Equal?(x=w242, y="Deslocamento_Retirada_por_Baixo") -> (x = y?=w238:bool)
                  n264 = Equal?(x=w242, y="Deslocamento_Retirada_por_Cima") -> (x = y?=w237:bool)
                  n265 = Build Array(w238, w237) -> (w239:bool[])
                  n266 = Boolean Array To Number(Boolean array=w239) -> (number=w236:u32)
                  n267 = case shown="0, Default" w236 {
                    tunnel: w379 -> [_ w389 w395]
                    tunnel: ["No Conf." w390 w394] -> w378
                    frame 0, Default {
                    }
                    frame 1 {
                      n268 = case shown="0, Default" w389 {
                        tunnel: ["No Conf." "C1" "C2"] -> w390
                        frame 0, Default {
                        }
                        frame 1 {
                        }
                        frame 2 {
                        }
                      }
                    }
                    frame 2 {
                      n269 = case shown="0, Default" w395 {
                        tunnel: ["No Conf." "C3" "C4"] -> w394
                        frame 0, Default {
                        }
                        frame 1 {
                        }
                        frame 2 {
                        }
                      }
                    }
                  }
                  "Configuração" <- w378
                  n270 = case shown="True" w310 {
                    frame False {
                    }
                    frame True {
                      # "Caso a válvula de aquisição\nseja acionada, a visualização \ndeve encerrar, para começar\na gravaçaao"
                      n271 = local write "Pontos No Gráfico"(10.0 ("POINTS IN GRAPH")) -> ()
                    }
                  }
                  n272 = Index Array(array=w349, index (row) #1=0 ("index (row)"), index (row) #2=1 ("index (row)"), index (row) #3=2 ("index (row)"), index (row) #4=3 ("index (row)"), index (row) #5=4 ("index (row)"), index (row) #6=5 ("index (row)")) -> (element #1=w341:dbl[], element #2=w340:dbl[], element #3=w339:dbl[], element #4=w338:dbl[], element #5=w337:dbl[], element #6=w336:dbl[])  [unwired: 6 in]
                  n273 = Index Array(array=w349, index (row) #1=7 ("index (row)"), index (row) #2=8 ("index (row)"), index (row) #3=9 ("index (row)"), index (row) #4=10 ("index (row)"), index (row) #5=11 ("index (row)"), index (row) #6=12 ("index (row)")) -> (element #1=w329:dbl[], element #2=w328:dbl[], element #3=w327:dbl[], element #4=w326:dbl[], element #5=w325:dbl[], element #6=w324:dbl[])  [unwired: 6 in]
                  n274 = Index Array(array=w349, index (row)=6) -> (element=w322:dbl[])  [unwired: 1 in]
                  n275 = Build Array(w341, w340, w339, w338, w337, w336, w329, w328, w327, w326, w325, w324, w322) -> (→"Gráfico":dbl[][])
                  n276 = local read "SAIR"() -> (w229:bool)
                  n277 = Index Array(array=w349, index (row) #1=0 ("index (row)"), index (row) #2=1 ("index (row)"), index (row) #3=2 ("index (row)"), index (row) #4=3 ("index (row)"), index (row) #5=4 ("index (row)"), index (row) #6=5 ("index (row)"), index (row) #7=6 ("index (row)"), index (row) #8=7 ("index (row)"), index (row) #9=8 ("index (row)"), index (row) #10=9 ("index (row)"), index (row) #11=10 ("index (row)"), index (row) #12=11 ("index (row)"), index (row) #13=12 ("index (row)")) -> (element #1=w382:dbl[], element #2=w373:dbl[], element #3=w361:dbl[], element #4=w360:dbl[], element #5=w359:dbl[], element #6=w358:dbl[], element #7=w357:dbl[], element #8=w356:dbl[], element #9=w355:dbl[], element #10=w354:dbl[], element #11=w353:dbl[], element #12=w352:dbl[], element #13=w351:dbl[])  [unwired: 13 in]
                  n278 = call-poly <vilib>:"Mean.vi"("X"=w382) -> ("mean"=w247:dbl)  [unwired: 1 out]
                  n279 = call-poly <vilib>:"Mean.vi"("X"=w373) -> ("mean"=w248:dbl)  [unwired: 1 out]
                  n280 = call-poly <vilib>:"Mean.vi"("X"=w361) -> ("mean"=w249:dbl)  [unwired: 1 out]
                  n281 = call-poly <vilib>:"Mean.vi"("X"=w360) -> ("mean"=w250:dbl)  [unwired: 1 out]
                  n282 = call-poly <vilib>:"Mean.vi"("X"=w359) -> ("mean"=w251:dbl)  [unwired: 1 out]
                  n283 = call-poly <vilib>:"Mean.vi"("X"=w358) -> ("mean"=w252:dbl)  [unwired: 1 out]
                  n284 = call-poly <vilib>:"Mean.vi"("X"=w357) -> ("mean"=w253:dbl)  [unwired: 1 out]
                  n285 = call-poly <vilib>:"Mean.vi"("X"=w356) -> ("mean"=w254:dbl)  [unwired: 1 out]
                  n286 = call-poly <vilib>:"Mean.vi"("X"=w355) -> ("mean"=w255:dbl)  [unwired: 1 out]
                  n287 = call-poly <vilib>:"Mean.vi"("X"=w354) -> ("mean"=w256:dbl)  [unwired: 1 out]
                  n288 = call-poly <vilib>:"Mean.vi"("X"=w353) -> ("mean"=w257:dbl)  [unwired: 1 out]
                  n289 = call-poly <vilib>:"Mean.vi"("X"=w352) -> ("mean"=w258:dbl)  [unwired: 1 out]
                  n290 = call-poly <vilib>:"Mean.vi"("X"=w351) -> ("mean"=w259:dbl)  [unwired: 1 out]
                  n291 = local write "C2-M corrente"(w250) -> ()
                  n292 = local write "C1-M corrente"(w247) -> ()
                  n293 = local write "C1-J corrente"(w248) -> ()
                  n294 = local write "P1 corrente"(w249) -> ()
                  n295 = local write "C2-J corrente"(w251) -> ()
                  n296 = local write "P2 corrente"(w252) -> ()
                  n297 = local write "Pfundo corrente"(w253) -> ()
                  n298 = local write "C3-M corrente"(w254) -> ()
                  n299 = local write "C3-J corrente"(w255) -> ()
                  n300 = local write "P3 corrente"(w256) -> ()
                  n301 = local write "C4-M corrente"(w257) -> ()
                  n302 = local write "C4-J corrente"(w258) -> ()
                  n303 = local write "P4 corrente"(w259) -> ()
                  n304 = Multiply(x=w253, y=0.25) -> (x*y=w266:dbl)
                  n305 = Multiply(x=w252, y=0.25) -> (x*y=w267:dbl)
                  n306 = Multiply(x=w257, y=0.25) -> (x*y=w262:dbl)
                  n307 = Multiply(x=w254, y=0.25) -> (x*y=w265:dbl)
                  n308 = Multiply(x=w255, y=0.25) -> (x*y=w264:dbl)
                  n309 = Multiply(x=w256, y=0.25) -> (x*y=w263:dbl)
                  n310 = Multiply(x=w258, y=0.25) -> (x*y=w261:dbl)
                  n311 = Multiply(x=w259, y=0.25) -> (x*y=w260:dbl)
                  n312 = Multiply(x=w250, y=0.25) -> (x*y=w269:dbl)
                  n313 = Multiply(x=w251, y=0.25) -> (x*y=w268:dbl)
                  n314 = Multiply(x=w248, y=0.25) -> (x*y=w271:dbl)
                  n315 = Multiply(x=w249, y=0.25) -> (x*y=w270:dbl)
                  n316 = Multiply(x=w247, y=0.25) -> (x*y=w272:dbl)
                  n317 = local write "C1-M"(w272) -> ()
                  n318 = local write "C1-J"(w271) -> ()
                  n319 = local write "P1"(w270) -> ()
                  n320 = local write "C2-M"(w269) -> ()
                  n321 = local write "C2-J"(w268) -> ()
                  n322 = local write "P2"(w267) -> ()
                  n323 = local write "Pfundo"(w266) -> ()
                  n324 = local write "C3-M"(w265) -> ()
                  n325 = local write "C3-J"(w264) -> ()
                  n326 = local write "P3"(w263) -> ()
                  n327 = local write "C4-M"(w262) -> ()
                  n328 = local write "C4-J"(w261) -> ()
                  n329 = local write "P4"(w260) -> ()
                  "led viewing" <- w231
                  "Visualização" <- w231
                }
                frame 2, 3 {
                  n330 = flat-sequence {
                    tunnel: [w474] -> w438
                    tunnel: [w473] -> w437
                    tunnel: w436 -> [w472]
                    tunnel: w435 -> [w471]
                    tunnel: w434 -> [w470]
                    tunnel: w431 -> [_]
                    tunnel: [w459] -> w430
                    tunnel: [w458] -> w429
                    tunnel: [w626] -> w432
                    tunnel: [w627] -> w433
                    tunnel: w429 -> [w626]
                    tunnel: w430 -> [w627]
                    frame #0 {
                      w444 = T4."Disabled and Grayed Out" ("Disabled")
                      # "adiciona o índice nome do arquivo"
                      # "Criação e edição dos nomes dos arquivos"
                      # "Aquisição de dados em paralelo da placa NI"
                      n331 = Current VI's Path() -> (path=w455:path)
                      n332 = Strip Path(path=w455) -> (stripped path=w454:path)  [unwired: 1 out]
                      n333 = property on="JW(m/s)" class="DigNum (strict)"("DisabledEnum"=w444) -> ()  [unwired: 2 in, 2 out]
                      n334 = property on="JK(m/s)" class="DigNum (strict)"("DisabledEnum"=w444) -> ()  [unwired: 2 in, 2 out]
                      n335 = property on="Gráfico" class="WFGraph (strict)"("DisabledEnum"=w444) -> ()  [unwired: 2 in, 2 out]
                      n336 = Build Path(base path=w454, name or relative path="PosProcessamento_UDP_NI\\data") -> (appended path=w456:path)
                      "data path" <- w456
                      n337 = local write "Finalizado"(FALSE ("Finalizado")) -> ()
                      n338 = Current VI's Path() -> (path=w466:path)
                      n339 = call "nome_arquivo_adq.vi"("caminho"=w456, "JW"="JW(N. Arquivo)", "JK"="JK(N. Arquivo)", "JG"="JG(N. Arquivo)") -> ("resulting string"=w446:string)  [unwired: 11 in]
                      n340 = local read "Quantidade de\narquivos adquiridos"() -> (w453:i64)
                      n341 = Strip Path(path=w466) -> (stripped path=w465:path)  [unwired: 1 out]
                      n342 = local read "TempoAquisicao"() -> (w445:dbl)
                      n343 = Build Path(base path=w465, name or relative path="Aquisicao_NI_paralelo.vi") -> (appended path=w464:path)
                      n344 = Open VI Reference(type specifier VI Refnum (for type only)=refnum<vi> refnum, vi path=w464, options=128) -> (vi reference=w463:refnum<vi>, error out=w460:errorcluster)  [unwired: 3 in]
                      n345 = local read "Frequência"() -> (w461:dbl)
                      n346 = Increment(x=w453) -> (x+1=w443:i64)
                      n347 = Format Into String(format string="%s%d%s", initial string=w446, "_" ("input 1"), w443, ".NI" ("substring (\"\")")) -> (resulting string=w452:string)  [unwired: 1 in, 1 out]
                      n348 = String To Path(string=w452) -> (path=w447:path)
                      n349 = flat-sequence {
                        frame #0 {
                          n350 = call <vilib>:"Beep.vi"("use system alert? (T)"=FALSE, "duration (msec)"=u32 50, "frequency (Hz)"=u32 528) -> ()  [unwired: 9 in]
                        }
                        frame #1 {
                          # "Aviso sonoro do inicio"
                          n351 = call <vilib>:"Beep.vi"("use system alert? (T)"=FALSE, "duration (msec)"=u32 50, "frequency (Hz)"=u32 665) -> ()  [unwired: 9 in]
                        }
                        frame #2 {
                          n352 = call <vilib>:"Beep.vi"("use system alert? (T)"=FALSE, "duration (msec)"=u32 50, "frequency (Hz)"=u32 790) -> ()  [unwired: 9 in]
                        }
                      }
                      n353 = call-by-ref "Start Asynchronous Call"(reference=w463, error in=w460, "rate"=w461, "Tempo de Aquisição"=w445, "file path (dialog if empty)"=w447, "task/channels in"=refnum<k21> "ADQUIRE" ("DAQmx Task Name")) -> ()  [unwired: 2 in, 5 out]
                      n354 = local write "Quantidade de\narquivos adquiridos"(w443) -> ()
                      n355 = while {
                        tunnel: ["SAIR"] -> w474
                        tunnel: [w489] -> w473
                        tunnel: w472 -> [w494]
                        tunnel: w471 -> [w492]
                        tunnel: w470 -> [w491]
                        tunnel: [errorcluster {"status"=FALSE, "code"=0, "source"=""} ("error out")] -> w459
                        tunnel: [refnum<k21> "ADQUIRE" ("task out")] -> w458
                        i -> [w493]
                        stop <- w495 stop-if-true
                        w485 = TRUE ("adq")
                        n356 = flat-sequence {
                          tunnel: w494 -> [w506]
                          tunnel: w492 -> [w529]
                          tunnel: w491 -> [w515]
                          frame #0 {
                            w507 = TRUE ("visu led")
                            (unwired) 3000
                            # "aréa de calculo para conversões e analise se os dados encontrados estão dentro de um padrão aceitavel"
                            # "Interpretação dos valores recebidos de outr\nPC e distribuido conforme a necessidade"
                            # "baseado nas configurações de valvulas abertas\né possível saber com qual tipo de configuração \nestá sendo trabalhado"
                            # "SIW-NC-CV-001 05"
                            # "SIK-CV-001 05 04"
                            # "SIT-CV-001 03"
                            # "ADQ 02"
                            # "SPW-WR-VEL 01"
                            # "SPK-WR-VEL 00"
                            n357 = local write "VALORES UDP"(w506) -> ()
                            n358 = Index Array(array=w506, index #1=0 ("index"), index #2=1 ("index"), index #3=2 ("index"), index #4=3 ("index"), index #5=4 ("index"), index #6=5 ("index"), index #7=10 ("index"), index #8=11 ("index")) -> (element #1=w559:string, element #2=w558:string, element #3=w557:string, element #4=w556:string, element #5=w555:string, element #6=w554:string, element #7=w500:string, element #8=w496:string)
                            n359 = local read "Pfundo corrente"() -> (w573:dbl)
                            n360 = local read "P1 corrente"() -> (w580:dbl)
                            n361 = local read "P2 corrente"() -> (w579:dbl)
                            n362 = local read "P3 corrente"() -> (w578:dbl)
                            n363 = local read "P4 corrente"() -> (w574:dbl)
                            n364 = call "CONVERSOR.vi"("String"=w559) -> ("float"=w530:dbl)  [unwired: 6 in, 3 out]
                            n365 = local write "JK(m/s)"(w530) -> ()
                            n366 = call "CONVERSOR.vi"("String"=w558) -> ("float"=w531:dbl)  [unwired: 6 in, 3 out]
                            n367 = local write "JW(m/s)"(w531) -> ()
                            n368 = call "CONVERSOR.vi"("String"=w557) -> ()  [unwired: 6 in, 4 out]
                            n369 = call "CONVERSOR.vi"("String"=w556) -> ("boolean"=w552:bool)  [unwired: 6 in, 3 out]
                            "Linha de Teste" <- w552
                            n370 = call "CONVERSOR.vi"("String"=w555) -> ("boolean"=w551:bool)  [unwired: 6 in, 3 out]
                            n371 = local write "SIK-CV-001"(w551) -> ()
                            n372 = call "CONVERSOR.vi"("String"=w554) -> ("boolean"=w550:bool)  [unwired: 6 in, 3 out]
                            n373 = local write "SIW-CV-001"(w550) -> ()
                            n374 = call "CONVERSOR.vi"("String"=w496) -> ("float"=w498:dbl)  [unwired: 6 in, 3 out]
                            "Pbarometro" <- w498
                            n375 = call "CONVERSOR.vi"("String"=w500) -> ("boolean"=w527:bool)  [unwired: 6 in, 3 out]
                            n376 = local write "SKS-NC-CV-006"(w527) -> ()
                            n377 = local read "arrayPbar"() -> (w499:dbl[])
                            n378 = call "variação_pressao_adq.vi"("P1(mA)"=w580, "P2(mA)"=w579, "P3(mA)"=w578, "P4(mA)"=w574, "PFUNDO(mA)"=w573, "JW(m/s)"=w531, "JK(m/s)"=w530, "Valores"=w529, "SIK-CV-001"=w551, "SIW-CV-001"=w550) -> ("P12/L12"=→"P12/L [Pa/m]":dbl, "P34/L34"=→"P34/L [Pa/m]":dbl, "P23/L23"=→"P23/L [Pa/m]":dbl, "P2(kPa)"=w534:dbl, "VALOR TEORICO"=w581:dbl, "P3(kPa)"=w533:dbl, "P1(kPa)"=w535:dbl, "P4(kPa)"=w532:dbl, "P1-P2G"=→"P1-P2 VERDE":bool, "P2-P3R"=→"P2-P3 RED":bool, "P2-P3G"=→"P2-P3 VERDE":bool, "P1-P2R"=→"P1-P2 RED":bool, "P3-P4G"=→"P3-P4 VERDE":bool, "P3-P4R"=→"P3-P4 RED":bool, "PFUNDO(kPa)"=w510:dbl)  [unwired: 3 in]
                            "P4(kPa)" <- w532
                            "P3(kPa)" <- w533
                            "P2(kPa)" <- w534
                            "P1(kPa)" <- w535
                            "Pfundo(kPa)" <- w510
                            n379 = Build Array (concatenate)(w499, w498) -> (w497:dbl[])
                            n380 = local write "arrayPbar"(w497) -> ()
                            n381 = local read "P1(kPa)"() -> (w505:dbl)
                            n382 = local read "P2(kPa)"() -> (w504:dbl)
                            n383 = local read "P3(kPa)"() -> (w503:dbl)
                            n384 = local read "P4(kPa)"() -> (w502:dbl)
                            n385 = call "check-up_adq.vi"("JK(m/s)"=w530, "JW(m/s)"=w531, "P4(kPa)"=w532, "P3(kPa)"=w533, "P2(kPa)"=w534, "P1(kPa)"=w535) -> ("OK 2 R"=→"OK2 R":bool, "OK 2 G"=→"OK2":bool, "OK RED"=→"Ok R":bool, "OK G"=→"Ok":bool)  [unwired: 2 in]
                            n386 = local read "ValoresEnviados"() -> (w514:T1)
                            n387 = Bundle By Name(cluster=w514, "Pfundo[kPa]"=w510, "DP_21"=w505, "DP_32"=w504, "DP_43"=w503, "DP_4Atm"=w502) -> (w516:T1)
                            n388 = case shown="True" w552 {
                              tunnel: w581 -> [_ w616]
                              frame False {
                                n389 = local write "Valor Teórico[Pa/m]"(nan) -> ()
                              }
                              frame True {
                                "Valor Teórico[Pa/m]" <- w616
                              }
                            }
                            n390 = invoke class="VI" method="Ctrl Val.Set"(reference=w515, "Control Name"="ValoresEnviados", "Value"=w514) -> ()  [unwired: 2 in, 5 out]
                            n391 = local write "ValoresEnviados"(w516) -> ()
                            n392 = case shown="True" TRUE {
                              tunnel: [w612 w614] -> w509
                              tunnel: [w597 w613] -> w508
                              tunnel: w531 -> [_ w614]
                              tunnel: w530 -> [_ w613]
                              frame False {
                                n393 = local read "Escala de Calibracao - SKM-FI-WF"() -> (w606:cluster{"Escala Max":dbl, "Escala Min":dbl})
                                n394 = local read "Entrada - SKM-FI-WF [CLP]"() -> (w604:dbl)
                                n395 = local read "SKM-FIC-KF_CORIOLI [kg/s]"() -> (w595:dbl)
                                n396 = local read "SKM-AI-KF_CORIOLI [kg/m³]"() -> (w594:dbl)
                                n397 = local read "Escala de Calibracao - SKM-FI-WF"() -> (w600:cluster{"Escala Max":dbl, "Escala Min":dbl})
                                n398 = Bundle By Name(cluster=w600, "Escala Max"=0.001805556, "Escala Min"=0.0 ("Escala Max")) -> (w601:cluster{"Escala Max":dbl, "Escala Min":dbl})
                                n399 = local write "Escala de Calibracao - SKM-FI-WF"(w601) -> ()
                                n400 = Unbundle By Name(w606) -> ("Escala Max"=w607:dbl, "Escala Min"=w605:dbl)
                                n401 = Divide(x=w595, y=w594) -> (x/y=w596:dbl)
                                n402 = Divide(x=w596, y=0.0005107051557) -> (x/y=w597:dbl)
                                n403 = Subtract(x=w607, y=w605) -> (x-y=w608:dbl)
                                n404 = Divide(x=w608, y=4096.0) -> (x/y=w609:dbl)
                                n405 = Multiply(x=w609, y=w604) -> (x*y=w610:dbl)
                                n406 = Add(x=w610, y=w605) -> (x+y=w611:dbl)
                                n407 = Divide(x=w611, y=0.0005107051557) -> (x/y=w612:dbl)
                              }
                              frame True {
                                # "devido a mudança do sistema para não ler valores do CLP , e sim de outro PC\nesse CASE deve ser mantido como TRUE até ordens de mudanças"
                              }
                            }
                            "JW(m/s)" <- w509
                            "JK(m/s)" <- w508
                            n408 = Index Array(array=w506, index #1=6 ("index"), index #2=7 ("index"), index #3=8 ("index"), index #4=9 ("index")) -> (element #1=w546:string, element #2=w545:string, element #3=w544:string, element #4=w541:string)
                            n409 = call "CONVERSOR.vi"("String"=w546) -> ("float"=w513:dbl)  [unwired: 6 in, 3 out]
                            n410 = call "CONVERSOR.vi"("String"=w545) -> ("float"=w512:dbl)  [unwired: 6 in, 3 out]
                            n411 = call "CONVERSOR.vi"("String"=w544) -> ("float"=w511:dbl)  [unwired: 6 in, 3 out]
                            n412 = call "CONVERSOR.vi"("String"=w541) -> ("float"=w540:dbl)  [unwired: 6 in, 3 out]
                            n413 = local write "JG(m/s)"(w540) -> ()
                            n414 = local write "SKM-FIC-KF-COR"(w512) -> ()
                            n415 = local write "SKM-AI-KF-COR"(w511) -> ()
                            n416 = local write "SKM-FI-WF"(w513) -> ()
                            n417 = local write "SIK-CV-001"(w551) -> ()
                            n418 = local write "SIW-CV-001"(w550) -> ()
                            n419 = local read "Aplicação"() -> (w519:string)
                            n420 = Build Array(w550, w551) -> (w572:bool[])
                            n421 = Boolean Array To Number(Boolean array=w572) -> (number=w521:u32)
                            n422 = Equal?(x=w519, y="Deslocamento_Retirada_por_Baixo") -> (x = y?=w523:bool)
                            n423 = Equal?(x=w519, y="Deslocamento_Retirada_por_Cima") -> (x = y?=w522:bool)
                            n424 = Build Array(w523, w522) -> (w524:bool[])
                            n425 = Boolean Array To Number(Boolean array=w524) -> (number=w520:u32)
                            n426 = case shown="2" w520 {
                              tunnel: w521 -> [_ w583 w589]
                              tunnel: ["No Conf." w584 w588] -> w518
                              frame 0, Default {
                              }
                              frame 1 {
                                n427 = case shown="1" w583 {
                                tunnel: ["No Conf." "C1" "C2"] -> w584
                                frame 0, Default {
                                }
                                frame 1 {
                                }
                                frame 2 {
                                }
                                }
                              }
                              frame 2 {
                                n428 = case shown="0, Default" w589 {
                                tunnel: ["No Conf." "C3" "C4"] -> w588
                                frame 0, Default {
                                }
                                frame 1 {
                                }
                                frame 2 {
                                }
                                }
                              }
                            }
                            n429 = local write "Configuração"(w518) -> ()
                            n430 = property on="Pontos No Gráfico" class="Knob (strict)"("DisabledEnum"=T4."Disabled and Grayed Out" ("Disabled")) -> ()  [unwired: 2 in, 2 out]
                            n431 = local write "led viewing"(w507) -> ()
                            n432 = local write "Visualização"(w507) -> ()
                          }
                          frame #1 {
                            n433 = Wait (ms)(milliseconds to wait=u32 1000) -> ()  [unwired: 1 out]
                          }
                        }
                        n434 = To Double Precision Float(number=w493) -> (double precision float=w488:dbl)
                        "Timer" <- w488
                        n435 = Greater Or Equal?(x=w488, y="TempoAquisicao") -> (x >= y?=w489:bool)
                        n436 = Compound Arithmetic op=OR(w489, "SAIR") -> (w495:bool)
                        "LED adquiri" <- w485
                        "Aquisição" <- w485
                      }
                      "arrayPbar" <- i32[] [] ("arrayPbar")
                    }
                    frame #1 {
                      n437 = flat-sequence {
                        frame #0 {
                          n438 = call <vilib>:"Beep.vi"("use system alert? (T)"=FALSE, "duration (msec)"=u32 50, "frequency (Hz)"=u32 1184) -> ()  [unwired: 9 in]
                        }
                        frame #1 {
                          n439 = Wait (ms)(milliseconds to wait=u32 1) -> ()  [unwired: 1 out]
                        }
                        frame #2 {
                          n440 = call <vilib>:"Beep.vi"("use system alert? (T)"=FALSE, "duration (msec)"=u32 50, "frequency (Hz)"=u32 790) -> ()  [unwired: 9 in]
                        }
                        frame #3 {
                          n441 = Wait (ms)(milliseconds to wait=u32 1) -> ()  [unwired: 1 out]
                        }
                        frame #4 {
                          n442 = call <vilib>:"Beep.vi"("use system alert? (T)"=FALSE, "duration (msec)"=u32 50, "frequency (Hz)"=u32 1056) -> ()  [unwired: 9 in]
                        }
                        frame #5 {
                          "Finalizado" <- TRUE ("Finalizado")
                        }
                      }
                      n443 = local read "Quantidade de\narquivos adquiridos"() -> (w622:i64)
                      n444 = Number To Decimal String(number=w622) -> (decimal integer string=w621:string)  [unwired: 1 in]
                      n445 = local read "data path"() -> (w624:path)
                      n446 = Concatenate Strings("Pbar\\Pbar_" ("string"), w621, ".txt" ("string")) -> (w620:string)
                      n447 = local read "arrayPbar"() -> (w625:dbl[])
                      n448 = Build Path(base path=w624, name or relative path=w620) -> (appended path=w619:path)
                      n449 = call-poly <vilib>:"Write Delimited Spreadsheet.vi"("file path (dialog if empty)"=w619, "1D data"=w625) -> ()  [unwired: 12 in, 2 out]
                    }
                  }
                }
              }
              n450 = Compound Arithmetic op=OR(w156, w157) -> (w158:bool)
              n451 = call <vilib>:"DAQmx Clear Task.vi"("task in"=w115, "error in"=w114) -> ("error out"=→"error out":errorcluster)  [unwired: 13 in]
              "DAQmx Task Name" <- w121
            }
            n452 = invoke class="VI" method="Abort VI"(reference=w89) -> ()  [unwired: 2 in, 3 out]
          }
          frame #2 {
            n453 = disable-structure shown="Enabled" {
              frame Disabled {
                # "salva em arquivo TXT tabela de\ndados com o nome ja montado"
                # "adiciona o índice nome do arquivo"
                # "Valores de entrada de velocidades para salvar no nome do arquivo\nVi também recebe o nome da configuração"
                # "Abre o diretório\"DADOS\" para armazenar os dados"
                # "Criação e edição dos nomes dos arquivos"
                n454 = Current VI's Path() -> (path=w706:path)
                n455 = Strip Path(path=w706) -> (stripped path=w705:path)  [unwired: 1 out]
                n456 = Build Path(base path=w705, name or relative path="Dados_Trifasico") -> (appended path=w696:path)
                n457 = call <vilib>:"Check if File or Folder Exists.vi"("path"=w696) -> ("file or folder exists?"=w698:bool, "dup path"=w697:path)  [unwired: 8 in, 1 out]
                n458 = case shown="True" w698 {
                  tunnel: w697 -> [w719 w720]
                  tunnel: [w718 w720] -> w695
                  frame False {
                    n459 = Create Folder(path (use dialog)=w719) -> (created path=w718:path)  [unwired: 2 in, 2 out]
                  }
                  frame True {
                  }
                }
                n460 = local read "JW(m/s)"() -> (w717:dbl)
                n461 = local read "JG(m/s)"() -> (w703:dbl)
                n462 = local read "JK(m/s)"() -> (w716:dbl)
                n463 = Number To Fractional String(number=w717, precision (6)=i16 2) -> (F-format string=w702:string)  [unwired: 2 in]
                n464 = Number To Fractional String(number=w716, precision (6)=i16 2) -> (F-format string=w701:string)  [unwired: 2 in]
                n465 = Number To Fractional String(number=w703, precision (6)=i16 2) -> (F-format string=w700:string)  [unwired: 2 in]
                n466 = call "nome_arquivo_adq.vi"("caminho"=w695, "JW"=w702, "JK"=w701, "JG"=w700) -> ("resulting string"=w699:string)  [unwired: 11 in]
                n467 = local read "Quantidade de\narquivos adquiridos"() -> (w713:i64)
                n468 = Current VI's Path() -> (path=w693:path)
                n469 = Increment(x=w713) -> (x+1=w707:i64)
                n470 = Format Into String(format string="%s%d%s", initial string=w699, "_" ("input 1"), w707, ".txt" ("substring (\"\")")) -> (resulting string=w709:string)  [unwired: 1 in, 1 out]
                n471 = String To Path(string=w709) -> (path=w708:path)
                n472 = local write "Quantidade de\narquivos adquiridos"(w707) -> ()
                n473 = Strip Path(path=w693) -> (stripped path=w694:path)  [unwired: 1 out]
                n474 = local read "Matriz"() -> (w684:dbl[][])
                n475 = Build Path(base path=w694, name or relative path="titulo.txt") -> (appended path=w691:path)
                n476 = Transpose 2D Array(2D array=w684) -> (transposed array=w689:dbl[][])
                n477 = call-poly <vilib>:"Read Delimited Spreadsheet.vi"("file path (dialog if empty)"=w691) -> ("first row"=w688:string[])  [unwired: 9 in, 5 out]
                n478 = Number To Fractional String(number=w689, precision (6)=i16 4) -> (F-format string=w687:string[][])  [unwired: 2 in]
                n479 = Build Array (concatenate)(w688, w687) -> (w686:string[][])
                n480 = call-poly <vilib>:"Write Delimited Spreadsheet.vi"("file path (dialog if empty)"=w708, "2D data"=w686) -> ()  [unwired: 12 in, 2 out]
              }
              frame Enabled {
              }
            }
          }
          frame #3 {
            w721 = FALSE ("Visualisa")
            # "botoões paara posição default"
            n481 = flat-sequence {
              frame #0 {
                # "para VI de comunicação com outro PC\nessa VI necessita se parada somento dessa meneira, de outro modo, dará erro"
                n482 = local read "reference out"() -> (w728:refnum<vi>)
                n483 = To Variant(anything=TRUE) -> (Variant=w725:variant)
                n484 = invoke class="VI" method="Ctrl Val.Set"(reference=w728, "Control Name"="STOP", "Value"=w725) -> ()  [unwired: 2 in, 5 out]
                n485 = Wait (ms)(milliseconds to wait=u32 500) -> ()  [unwired: 1 out]
              }
            }
            n486 = global write "comunicacao.vi" "comunicacao"(TRUE ("comunicacao")) -> ()
            n487 = local write "COMEÇAR"(w721) -> ()
            n488 = local write "Visualizar"(w721) -> ()
            n489 = local write "LED adquiri"(w721) -> ()
            n490 = local write "P1-P2 VERDE"(w721) -> ()
            n491 = local write "P1-P2 RED"(w721) -> ()
            n492 = local write "P2-P3 VERDE"(w721) -> ()
            n493 = local write "P2-P3 RED"(w721) -> ()
            n494 = local write "P3-P4 VERDE"(w721) -> ()
            n495 = local write "P3-P4 RED"(w721) -> ()
            n496 = local write "led viewing"(w721) -> ()
            n497 = local write "OK2"(w721) -> ()
            n498 = local write "OK2 R"(w721) -> ()
            n499 = local write "Ok"(w721) -> ()
            n500 = local write "Ok R"(w721) -> ()
            n501 = local write "Aquisição"(w721) -> ()
            n502 = local write "Aquisição Automática"(w721) -> ()
            n503 = local write "Visualização"(w721) -> ()
            n504 = local write "comunica funcionando"(w721) -> ()
            n505 = local read "SAIR"() -> (w723:bool)
          }
        }
      }
    }
    frame #1 {
      # "Como a VI \"abre aplicacção\" é a ultima a ser fechada\napós o termino do addquiri, será aberto ela denovo \npara caso o usurário deseje realizar outra aquisição \ncom outra aplicação, ou alterar alguma configuração"
      # "fecha VI"
      n506 = property class="VI"(error in=w730, "Front Panel.Open"=TRUE ("Front Panel Window:Open")) -> ()  [unwired: 1 in, 2 out]
      n507 = Current VI's Path() -> (path=w737:path)
      n508 = Strip Path(path=w737) -> (stripped path=w731:path)  [unwired: 1 out]
      n509 = Build Path(base path=w731, name or relative path="abre_aplicacao_adq.vi") -> (appended path=w735:path)
      n510 = Open VI Reference(vi path=w735) -> (vi reference=w734:refnum<vi>)  [unwired: 5 in, 1 out]
      n511 = invoke class="VI" method="Run VI"(reference=w734, "Wait until done"=FALSE ("Wait Until Done"), "Auto Dispose Ref"=FALSE ("Auto Dispose Reference")) -> ()  [unwired: 2 in, 5 out]
    }
  }
